vi "hex_whitespace_in_string.vi"(11 "string":string) -> (3 "hexed_string":string)   [LabVIEW 2020]
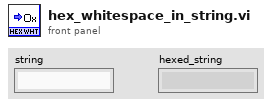
[diagram p1: front panel]
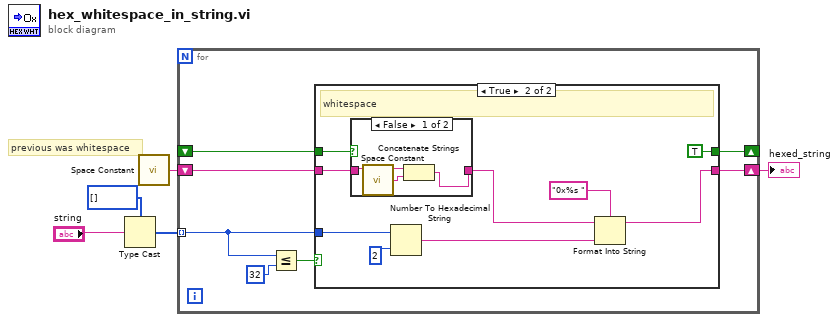
[diagram p0: block diagram]
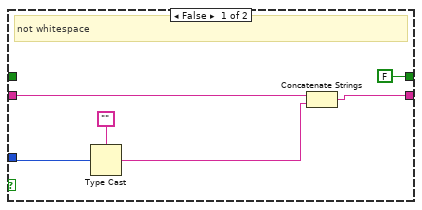
[diagram p2: hidden frame]
diagram:
  # "previous was whitespace"
  n1 = Type Cast(type=u8[] [], x="string") -> (*(type *) &x=w3:u8[])
  n2 = call <vilib>:"Space Constant.vi"() -> ("String"=w1:string)
  n3 = for {
    tunnel: w3 -> [w8] mode=indexing
    shift-right: [w12] -> w2
    shift-left: w1 -> [w11]
    shift-right: [w7] -> _
    shift-left: _ -> [w6]
    n4 = Less Or Equal?(x=w8, y=u8 32) -> (x <= y?=w9:bool)
    n5 = case shown="True" w9 {
      tunnel: [w14 w24] -> w12
      tunnel: w11 -> [w16 w20]
      tunnel: w8 -> [w18 w23]
      tunnel: [FALSE TRUE] -> w7
      tunnel: w6 -> [_ w21]
      frame False {
        # "not whitespace"
        n6 = Type Cast(type="", x=w18) -> (*(type *) &x=w15:string)
        n7 = Concatenate Strings(w16, w15) -> (w14:string)
      }
      frame True {
        # "whitespace"
        n8 = case shown="False" w21 {
          tunnel: w20 -> [w30 w31]
          tunnel: [w28 w31] -> w19
          frame False {
            n9 = call <vilib>:"Space Constant.vi"() -> ("String"=w29:string)
            n10 = Concatenate Strings(w30, w29) -> (w28:string)
          }
          frame True {
          }
        }
        n11 = Number To Hexadecimal String(1:i16 2 ("width (-)"), 2:w23) -> (0:w26:string)
        n12 = Format Into String(format string="0x%s ", initial string=w19, w26) -> (resulting string=w24:string)  [unwired: 1 in, 1 out]
      }
    }
  }
  "hexed_string" <- w2
